vi "Robot Main.vi"() -> ()   [LabVIEW 2012]
doc: "This VI imlements the framework and scheduler for your robotics program. It should not be necessary to modify the framework. You are expected to add your code to the VIs called from Robot Main, the ones located in the Team Code within the project."
uses:
  <vilib>/Rock Robotics/WPI/Camera/WPI_CameraImageSize.ctl
  Inputs_All.ctl
  Flywheel/Sensor_Inputs_FlyWheel.ctl
  tankdrive/Input_Sensors_Drive.ctl
  Conveyor/Sensor_Input_Conveyor.ctl
  Conveyor/Sensor_Input_ConveyorV2.ctl
  Turret/Inputs_Sensors_Turret.ctl
  Inputs_Camera.ctl
  Outputs_All.ctl
  Flywheel/Outputs_Flywheel.ctl
  tankdrive/Output_Wheel_Speeds.ctl
  Conveyor/Conveyor_outputs.ctl
  Conveyor/Conveyor module state.ctl
  Conveyor/Conveyor_outputsV2.ctl
  Conveyor/3-Ball-Conveyor_Module_State.ctl
  Conveyor/T_Roller module state.ctl
  Turret/Outputs_Turret.ctl
  Roller/Outputs_Roller.ctl
  Bridge Tipper/Outputs_Tipper.ctl
  <vilib>/Rock Robotics/WPI/DriverStation/WPI_DriverStationRobotMode.ctl
  <vilib>/Platform/TimedLoop/XDataNode/timing_clust.ctl
  <vilib>/Platform/TimedLoop/XDataNode/nitl_modes.ctl
  <vilib>/Platform/TimedLoop/XDataNode/wakeup.ctl
  Robot Global Data.vi
  <vilib>/Platform/TimedLoop/XDataNode/XDataNode.xnode
  <vilib>/Platform/TimedLoop/XDataNode/XDNodeRunTimeDep.lvlib
panel:
  out "Camera Inputs":T1
  out "Robot Mode":T2
  in  "Take Pics":bool
  out "dt":u32=50
  out "OutputsCluster":T3
  out "Sensor Inputs":T14
  in  "Image Size":T20=enum."320x240"
  in  "Enable Vision":bool=TRUE
  in  "Finish":bool
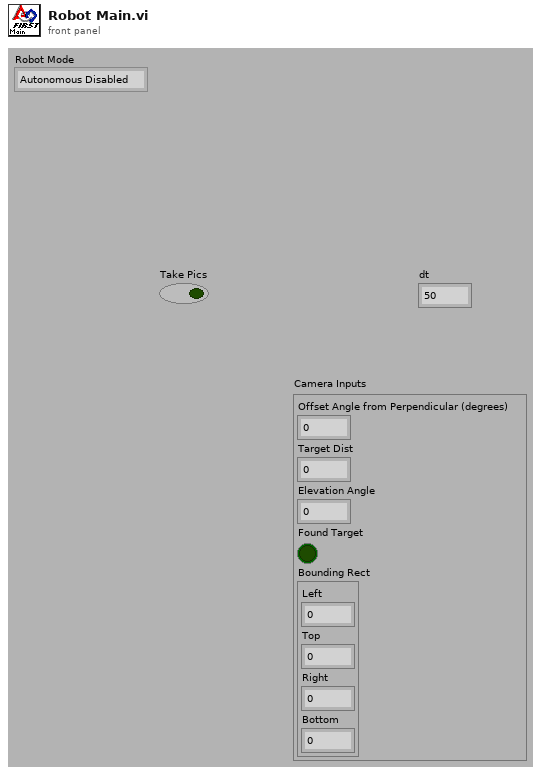
[diagram p1: front panel]
types:
  T1 = typedef "Inputs_Camera.ctl" = cluster{"Offset Angle from Perpendicular (degrees)":dbl, "Target Dist":dbl, "Elevation Angle":dbl, "Found Target":bool, "Bounding Rect":cluster{"Left":dbl, "Top":dbl, "Right":dbl, "Bottom":dbl}}
  T2 = typedef "WPI_DriverStationRobotMode.ctl" = enum16{"Autonomous Disabled", "Autonomous Enabled", "Teleop Disabled", "Teleop Enabled", "Timeout", "Finish"}
  T3 = typedef "Outputs_All.ctl" = cluster{"Flywheel Outputs":T4, "Drive Outputs":T5, "Conveyor Outputs":T6, "Conveyor Outputs 2":T8, "Turret Outputs":T11, "Roller Outputs":T12, "Bridge Tipper Outputs":T13}
  T4 = typedef "Outputs_Flywheel.ctl" = cluster{"Wheel Speed":dbl}
  T5 = typedef "Output_Wheel_Speeds.ctl" = cluster{"Front Left Speed":dbl, "Front Right Speed":dbl, "Back Left Speed":dbl, "Back Right Speed":dbl}
  T6 = typedef "Conveyor_outputs.ctl" = cluster{"Bottom Conveyor Speed":dbl, "Top Conveyor Speed":dbl, "Bottom Conveyor State":T7, "Top Conveyor State":T7, "Accepting Balls":bool, "Number of Balls":i32}
  T7 = typedef "Conveyor module state.ctl" = enum16{"No Ball", "Has Ball", "Ball Below Hold", "Ball Above Hold", "Outputting Ball", "Reset"}
  T8 = typedef "Conveyor_outputsV2.ctl" = cluster{"Accepting Balls":bool, "Number of Balls":i32, "Conveyor State":T9, "Top Roller State":T10, "Top Roller":dbl, "Conveyor":dbl}
  T9 = typedef "3-Ball-Conveyor_Module_State.ctl" = enum16{"No Balls", "Collecting Ball", "Holding 1", "Pushing Ball Out", "Holding 2", "Lowering Ball", "Reset", "Disabled"}
  T10 = typedef "T_Roller module state.ctl" = enum16{"Reset", "Disabled", "Waiting for Ball", "Holding", "Ball not far enough", "Ball too far", "Firing"}
  T11 = typedef "Outputs_Turret.ctl" = cluster{"Desired Position":dbl, "Is Reset":bool, "Target In Deadzone":bool}
  T12 = typedef "Outputs_Roller.ctl" = cluster{"Front Roller":dbl}
  T13 = typedef "Outputs_Tipper.ctl" = cluster{"Speed":dbl}
  T14 = typedef "Inputs_All.ctl" = cluster{"Inputs_FlyWheel":T15, "Drive Inputs":T16, "Conveyor Inputs":T17, "ConveyorV2 Inputs":T18, "Turret Inputs":T19, "Camera Inputs":T1}
  T15 = typedef "Sensor_Inputs_FlyWheel.ctl" = cluster{"Speed":dbl, "Target Distance":dbl}
  T16 = typedef "Input_Sensors_Drive.ctl" = cluster{"Left Front Speed":dbl, "Right Front Speed":dbl, "Left Back Speed":dbl, "Right Back Speed":dbl}
  T17 = typedef "Sensor_Input_Conveyor.ctl" = cluster{"Top Ball Detector Count":i32, "Bottom Ball Detector Count":i32, "Shooter Ball Detector Count":i32}
  T18 = typedef "Sensor_Input_ConveyorV2.ctl" = cluster{"Grab Ball Detector Count":i32, "Bottom Ball Detector Count":i32, "Top In Place Ball Detector Count":i32, "Top Too Far Ball Detector Count":i32, "Top Not Far Enough":i32}
  T19 = typedef "Inputs_Sensors_Turret.ctl" = cluster{"At Minimum Angle":bool, "At Maximum Angle":bool, "Camera Position Offset":dbl, "Found Target?":bool, "Position Encoder":dbl}
  T20 = typedef "WPI_CameraImageSize.ctl" = enum16{"640x480", "320x240", "160x120"}
  T21 = typedef "XDNodeRunTimeDep.lvlib/timing_clust.ctl" = cluster{"Expected End [f-1]":u64, "Actual End [f-1]":u64, "Finished Late? [f-1]":bool, "Expected End [i-1]":u64, "Actual End [i-1]":u64, "Finished Late? [i-1]":bool, "Expected Start [i]":u64, "Actual Start [i]":u64, "Expected Start [f]":u64, "Actual Start [f]":u64, "Source Name":string, "Structure Name":string, "Period":i64, "Deadline":i64, "Offset":i64, "Start":i64, "Priority":i32, "Timeout":i32, "Mode":T22, "Wakeup Reason":T23, "Error":errorcluster, "Source Type":string, "Secondary Source Type":string, "Global End Time":u64, "Global Start Time":u64, "Frame Duration":u64, "Iteration Duration":u64, "Assigned CPU":i32, "I/O Scan Engine Mode":u32}
  T22 = typedef "XDNodeRunTimeDep.lvlib/nitl_modes.ctl" = enum32{"No Change", "Process missed periods, maintain original phase", "Discard missed periods, maintain original phase", "Process missed periods, ignore original phase", "Discard missed periods, ignore original phase"}
  T23 = typedef "XDNodeRunTimeDep.lvlib/wakeup.ctl" = enum32{"Normal", "Aborted", "Asynchronous wakeup", "Timing source error", "Timed loop error", "Timeout"}
  T24 = typedef "WPI_CameraDevRef.ctl" = cluster{"Camera Address":string, "CameraStatus":errorcluster, "Acquire Image Notifier":refnum<notifier>}
  T25 = cluster{"Left":dbl, "Top":dbl, "Right":dbl, "Bottom":dbl}
  T26 = typedef "WPI_DriverStationMatch Info.ctl" = cluster{"Autonomous Elapsed Seconds":dbl, "TeleOp Elapsed Seconds":dbl, "Disabled Elapsed Seconds":dbl, "Visited Autonomous":bool, "Visited TeleOp":bool, "Visited Disabled":bool, "Autonomous Settings":cluster{"Autonomous Style":enum16{"Iterative", "Independent"}, "VI Refnum":refnum<vi>}}
  T27 = typedef "WPI_DriverStationDerivedRobotMode.ctl" = enum16{"Init", "Execute", "Stop"}
  T28 = typedef "Command_Inputs.ctl" = cluster{"Drive Command Inputs":T29, "Conveyor Command Inputs":T30, "Turret Command Inputs":T31, "Tipper Command Inputs":T32, "Dasboard Controls":T33, "Roller Commands":T34, "Flywheel Commands":T35}
  T29 = typedef "Input_Commands_Drive.ctl" = cluster{"Tank Left Command":dbl, "Tank Right Command":dbl, "Arcade Forward Command":dbl, "Arcade Right Comand":dbl, "Drive Slowly":bool, "Auto-align tipper":bool}
  T30 = typedef "Input_Command_Conveyor.ctl" = cluster{"Shoot a Ball":bool, "Reset":bool, "Enable Conveyor":bool}
  T31 = typedef "Inputs_Commands_Turret.ctl" = cluster{"Reset Turret":bool, "User Position Change Command":dbl, "Aim with camera":bool}
  T32 = typedef "Inputs_Tipper.ctl" = cluster{"Tipper Comand":dbl}
  T33 = typedef "Dashboard Controls.ctl" = cluster{"Joystick Right/Left":dbl, "Joystick Up/Down":dbl, "Use top camera":bool}
  T34 = typedef "Input_Commands_Roller.ctl" = cluster{"Enable Front Roller":bool}
  T35 = typedef "Input_Commands_Flywheel.ctl" = cluster{"Key Mode":bool, "Layup Mode":bool, "Flywheel Speed Offset":dbl, "Distance Mode":bool, "Lob Mode":bool, "Reset":bool, "Reverse (slow)":bool}
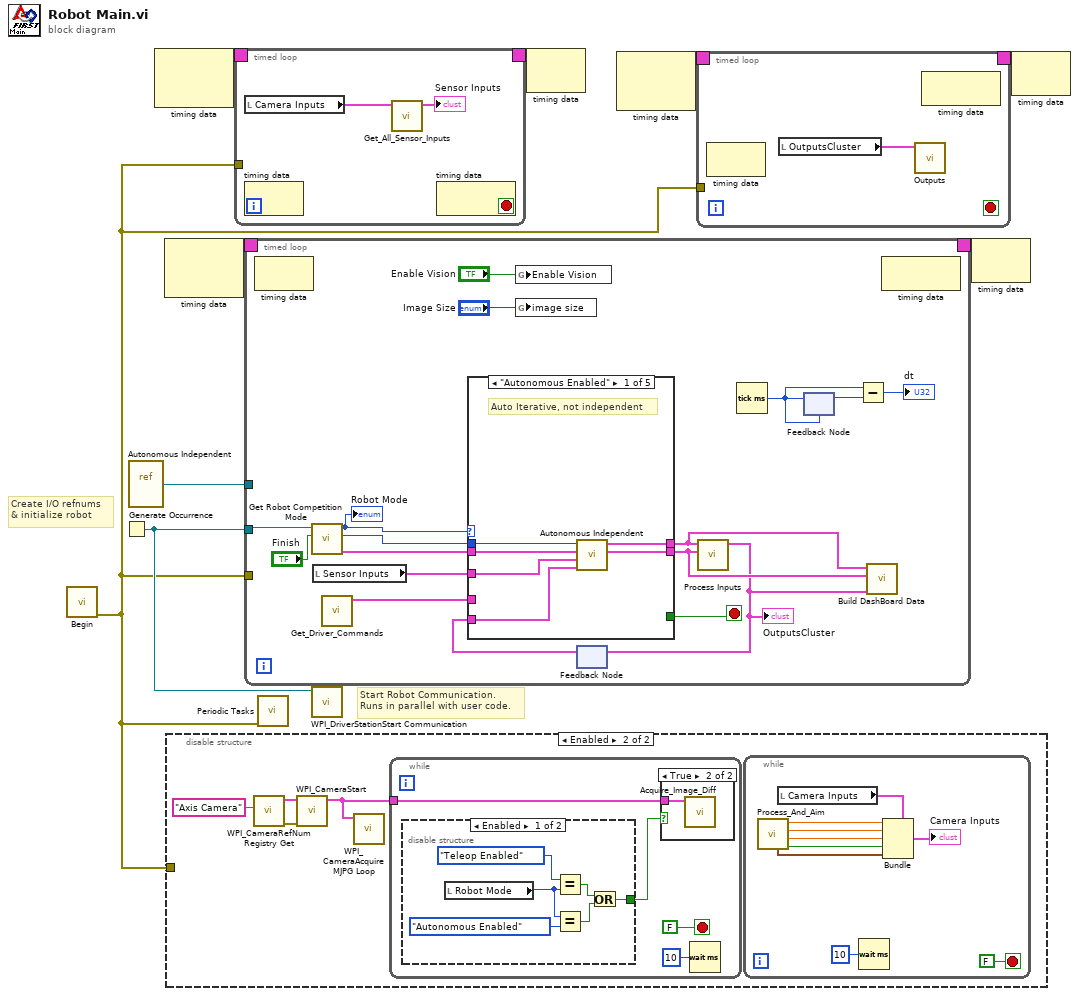
[diagram p0: block diagram]
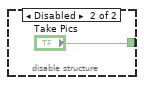
[diagram p3: hidden frame]
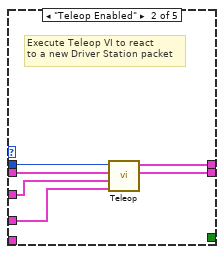
[diagram p5: hidden frame]
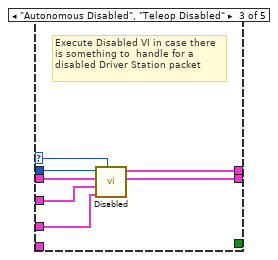
[diagram p6: hidden frame]
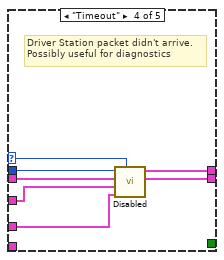
[diagram p7: hidden frame]
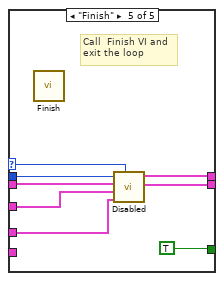
[diagram p8: hidden frame]
diagram:
  # "Create I/O refnums\n& initialize robot"
  # "Start Robot Communication.\nRuns in parallel with user code."
  n1 = call "Begin.vi"() -> ("No error"=w1:errorcluster)  [unwired: 11 in]
  n2 = Generate Occurrence() -> (w9:refnum<k4>)
  n3 = vi-ref "Autonomous Independent.vi"() -> (w8:refnum<vi>)
  n4 = node-c288() -> (w5:T21)  [unwired: 2 in]
  n5 = node-c288() -> (w7:T21)  [unwired: 2 in]
  n6 = disable-structure shown="Enabled" {
    disable-tunnel: w1 -> [_ _]
    frame Disabled {
    }
    frame Enabled {
      n7 = call <vilib>:"WPI_CameraRefNum Registry Get.vi"("refnum name"="Axis Camera") -> ("error out"=w11:errorcluster, "CameraDevRef"=w12:T24)  [unwired: 9 in]
      n8 = call <vilib>:"WPI_CameraStart.vi"("error in (no error)"=w11, "CameraDevRef"=w12) -> ("CameraDevRef Out"=w13:T24)  [unwired: 8 in, 1 out]
      n9 = call <vilib>:"WPI_CameraAcquire MJPG Loop.vi"("CameraDevRef"=w13) -> ()  [unwired: 11 in]
      n10 = while {
        tunnel: w13 -> [w26]
        stop <- FALSE stop-if-true
        n11 = disable-structure shown="Enabled" {
          disable-tunnel: [w27 "Take Pics"] -> w23
          frame Enabled {
            n12 = local read "Robot Mode"() -> (w31:T2)
            n13 = Equal?(x=WPI_DriverStationRobotMode."Teleop Enabled", y=w31) -> (x = y?=w29:bool)
            n14 = Equal?(x=w31, y=WPI_DriverStationRobotMode."Autonomous Enabled") -> (x = y?=w28:bool)
            n15 = Or(x=w29, y=w28) -> (x .or. y?=w27:bool)
          }
          frame Disabled {
          }
        }
        n16 = case shown="True" w23 {
          tunnel: w26 -> [_ w34]
          frame False {
          }
          frame True {
            n17 = call "Acquire_Image_Diff.vi"("CameraDevRef"=w34) -> ()  [unwired: 11 in]
          }
        }
        n18 = Wait (ms)(milliseconds to wait=u32 10) -> ()  [unwired: 1 out]
      }
      n19 = while {
        stop <- FALSE stop-if-true
        n20 = call "Process_And_Aim.vi"() -> ("Found Target"=w16:bool, "Elevation Angle"=w18:dbl, "Target Dist"=w19:dbl, "Offset Angle From Perpendicular"=w20:dbl, "Bounding Rect"=w17:T25)  [unwired: 7 in]
        n21 = local read "Camera Inputs"() -> (w21:T1)
        n22 = Wait (ms)(milliseconds to wait=u32 10) -> ()  [unwired: 1 out]
        n23 = Bundle(cluster=w21, "Offset Angle from Perpendicular (degrees)"=w20, "Target Dist"=w19, "Elevation Angle"=w18, "Found Target"=w16, "Bounding Rect"=w17) -> (→"Camera Inputs":T1)
      }
    }
  }
  n24 = timed-loop {
    timing: w5 -> [_]
    timing-out: [_] -> w4
    tunnel: w1 -> [_]
    stop <- _ stop-if-true
    n25 = local read "Camera Inputs"() -> (w35:T1)
    n26 = node-c288() -> ()  [unwired: 1 in, 1 out]
    n27 = call "Get_All_Sensor_Inputs.vi"("Camera Inputs"=w35) -> ("Input_Sensors"=→"Sensor Inputs":T14)  [unwired: 10 in]
    n28 = node-c288() -> ()  [unwired: 1 in, 1 out]
  }
  n29 = timed-loop {
    tunnel: w9 -> [w53]
    tunnel: w1 -> [_]
    tunnel: w8 -> [_]
    timing: w7 -> [_]
    timing-out: [_] -> w6
    stop <- w50 stop-if-true
    n30 = node-c288() -> ()  [unwired: 1 in, 1 out]
    n31 = call "Get Robot Competition Mode.vi"("Finish"="Finish", "DS Occurrence"=w53) -> ("Match Info out"=w51:T26, "Call Context"=w55:T27, "Robot Mode"=w54:T2)  [unwired: 7 out]
    "Robot Mode" <- w54
    n32 = local read "Sensor Inputs"() -> (w47:T14)
    n33 = call "Get_Driver_Commands.vi"() -> ("Driver Command_Inputs"=w43:T28)  [unwired: 11 in]
    n34 = global write "Robot Global Data.vi" "Enable Vision"("Enable Vision") -> ()
    n35 = global write "Robot Global Data.vi" "image size"("Image Size") -> ()
    n36 = feedback #1() -> (w39:T3)  [unwired: 1 in]
    n37 = case shown="\"Autonomous Enabled\"" w54 {
      selector: w54 -> [_ _ w74 w78 w88]
      tunnel: w55 -> [w63 w69 w76 w81 w87]
      tunnel: w51 -> [w62 w68 w75 w80 w86]
      tunnel: [_ _ _ _ TRUE] -> w50
      tunnel: w47 -> [w61 w67 w71 w79 w85]
      tunnel: w43 -> [_ w66 w70 w77 w84]
      tunnel: [w60 w65 w73 w83 w90] -> w42
      tunnel: [w59 w64 w72 w82 w89] -> w41
      tunnel: w39 -> [w58 _ _ _ _]
      frame "Autonomous Enabled" {
        # "Auto Iterative, not independent"
        n38 = call "Autonomous Independent.vi"("Previous Outputs"=w58, "Sensor Inputs"=w61, "Match Info"=w62, "Call Context"=w63) -> ("Auto Commands"=w59:T28, "Sensor Inputs (out)"=w60:T14)  [unwired: 6 in]
      }
      frame "Teleop Enabled" {
        # "Execute Teleop VI to react\nto a new Driver Station packet"
        n39 = call "Teleop.vi"("Driver Command Inputs"=w66, "Sensor Inputs"=w67, "Match Info"=w68, "Call Context"=w69) -> ("Commands"=w64:T28, "Sensor Inputs"=w65:T14)  [unwired: 6 out]
      }
      frame "Autonomous Disabled", "Teleop Disabled" {
        # "Execute Disabled VI in case there\nis something to  handle for a\ndisabled Driver Station packet"
        n40 = call "Disabled.vi"("Robot Mode"=w74, "Driver Command_Inputs"=w70, "Sensor Inputs (in)"=w71, "Match Info"=w75, "Call Context"=w76) -> ("Disabled Commands"=w72:T28, "Sensor Inputs (out)"=w73:T14)  [unwired: 5 out]
      }
      frame "Timeout" {
        # "Driver Station packet didn't arrive.\nPossibly useful for diagnostics"
        n41 = call "Disabled.vi"("Robot Mode"=w78, "Driver Command_Inputs"=w77, "Sensor Inputs (in)"=w79, "Match Info"=w80, "Call Context"=w81) -> ("Disabled Commands"=w82:T28, "Sensor Inputs (out)"=w83:T14)  [unwired: 5 out]
      }
      frame "Finish" {
        # "Call  Finish VI and\nexit the loop"
        n42 = call "Finish.vi"() -> ()  [unwired: 1 in, 7 out]
        n43 = call "Disabled.vi"("Robot Mode"=w88, "Driver Command_Inputs"=w84, "Sensor Inputs (in)"=w85, "Match Info"=w86, "Call Context"=w87) -> ("Disabled Commands"=w89:T28, "Sensor Inputs (out)"=w90:T14)  [unwired: 5 out]
      }
    }
    n44 = call "Process Inputs.vi"("Command Inputs"=w41, "Sensor Inputs"=w42) -> ("OutputsCluster"=w40:T3)  [unwired: 9 in]
    "OutputsCluster" <- w40
    n45 = feedback-in #1(w40) -> ()
    n46 = Tick Count (ms)() -> (millisecond timer value=w45:u32)
    n47 = feedback-in #2(w45) -> ()
    n48 = feedback #2(w45) -> (w46:u32)
    n49 = Subtract(x=w45, y=w46) -> (x-y=→"dt":u32)
    n50 = call "Build DashBoard Data.vi"("OutputsCluster"=w40, "Command_Inputs"=w41, "Sensor_Inputs"=w42) -> ()  [unwired: 9 out]
    n51 = node-c288() -> ()  [unwired: 1 in, 1 out]
  }
  n52 = call "Periodic Tasks.vi"("error in"=w1) -> ()  [unwired: 1 in, 10 out]
  n53 = call <vilib>:"WPI_DriverStationStart Communication.vi"("occurrence"=w9) -> ()  [unwired: 11 out]
  n54 = node-c288(w4) -> ()  [unwired: 1 out]
  n55 = node-c288() -> (w3:T21)  [unwired: 2 in]
  n56 = timed-loop {
    timing: w3 -> [_]
    timing-out: [_] -> w2
    tunnel: w1 -> [_]
    stop <- _ stop-if-true
    n57 = node-c288() -> ()  [unwired: 1 in, 1 out]
    n58 = local read "OutputsCluster"() -> (w92:T3)
    n59 = call "Outputs.vi"("OutputsCluster"=w92) -> ()  [unwired: 11 in]
    n60 = node-c288() -> ()  [unwired: 1 in, 1 out]
  }
  n61 = node-c288(w6) -> ()  [unwired: 1 out]
  n62 = node-c288(w2) -> ()  [unwired: 1 out]
